vi "2 IPs same subnet check.vi"(9 "IP2":string, 10 "subnetmask":string, 11 "IP1":string) -> (2 "IP1 net address":u32, 3 "same subnet?":bool)   [LabVIEW 2020]
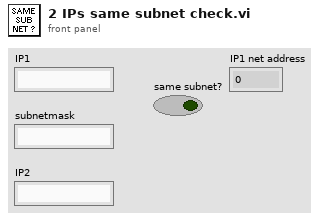
[diagram p1: front panel]
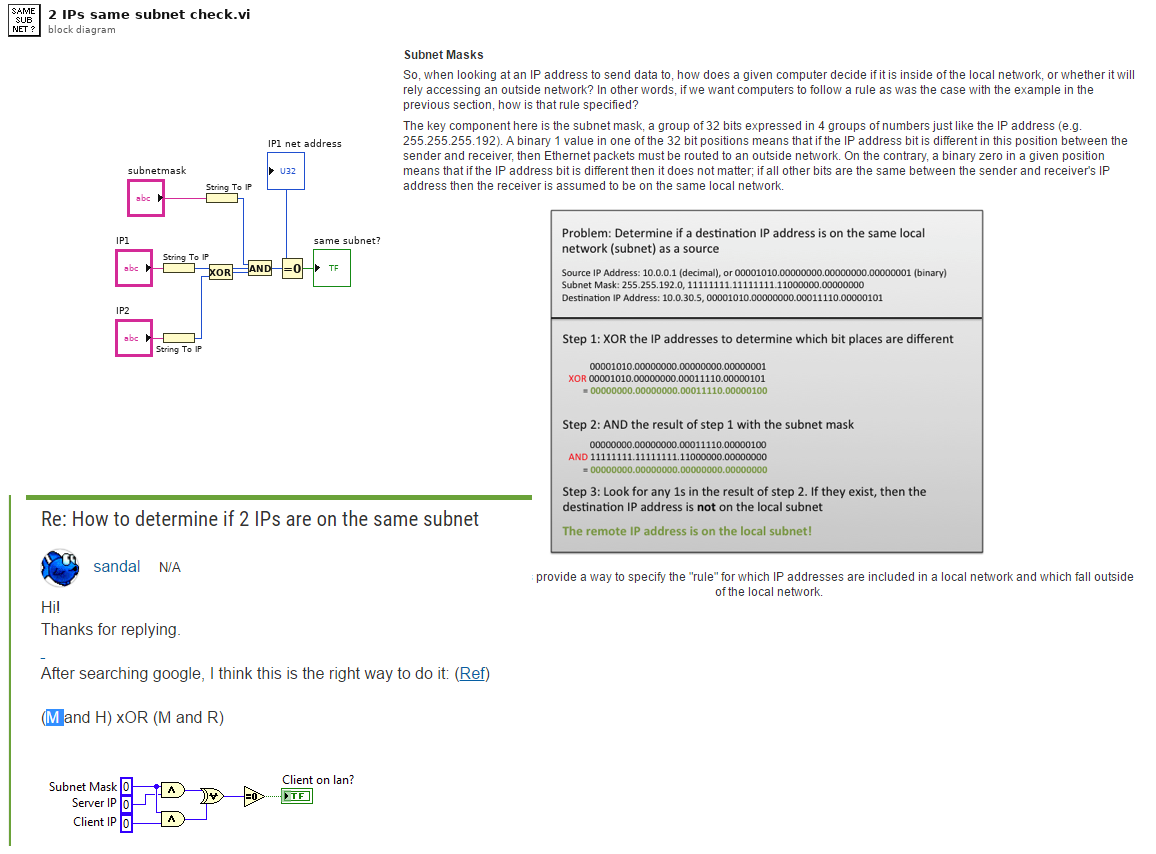
[diagram p0: block diagram]
diagram:
  n1 = String To IP(1:"IP1") -> (0:w4:u32)
  "IP1 net address" <- w4
  n2 = String To IP(1:"IP2") -> (0:w5:u32)
  n3 = Exclusive Or(1:w5, 2:w4) -> (0:w7:u32)
  n4 = String To IP(1:"subnetmask") -> (0:w6:u32)
  n5 = And(x=w6, y=w7) -> (x .and. y?=w8:u32)
  n6 = Equal To 0?(x=w8) -> (x = 0?=→"same subnet?":bool)
